vi "tsc-Show Control Settings--dialog.vi"(10 "VI Refnum":refnum<vi>) -> ()   [LabVIEW 2021]
doc: "This VI will be the user interface function for the Quick Drop action - it will list all controls on the front panel along with their UI Theme Levels and Boolean Types. This will be populated before showing its front panel and will give the user faster access to edit all controls on the front panel.\n\n->If there are any changes made and \"Apply\" is selected, it will apply the updated tags and save the VI\n->If Cancel is selected, the updates made will not be implemented\n\n<b>Code Developed By:</b>\nTechnology Service Corporation\n1983 S Liberty Drive\nBloomington, IN 47403\nPhone: 812 558-7100\nwww.tsc.com/atcs\n\nDeveloper:\nDaniel Coons"
uses:
  <vilib>/Utility/traverseref.llb/VI Scripting - Traverse.lvlib
  <vilib>/Utility/traverseref.llb/TRef TravTarget.ctl
  control info.ctl
  user32.dll
panel:
  out "header":bool
  in  "Cancel":bool
  in  "Apply":bool
  in  "control info":T1[](array[typedef]) {"Boolean Type" items=["Undefined", "N/A", "Outline", "No-Outline", "Tonal", "Filled", "Transparent", "FAB", "Elevated"]; "UI Theme Level" items=["Undefined", "N/A", "Primary", "Secondary", "Tertiary", "Error", "Primary Fixed", "Secondary Fixed", "Tertiary Fixed", "Label Only", "No Change"]}
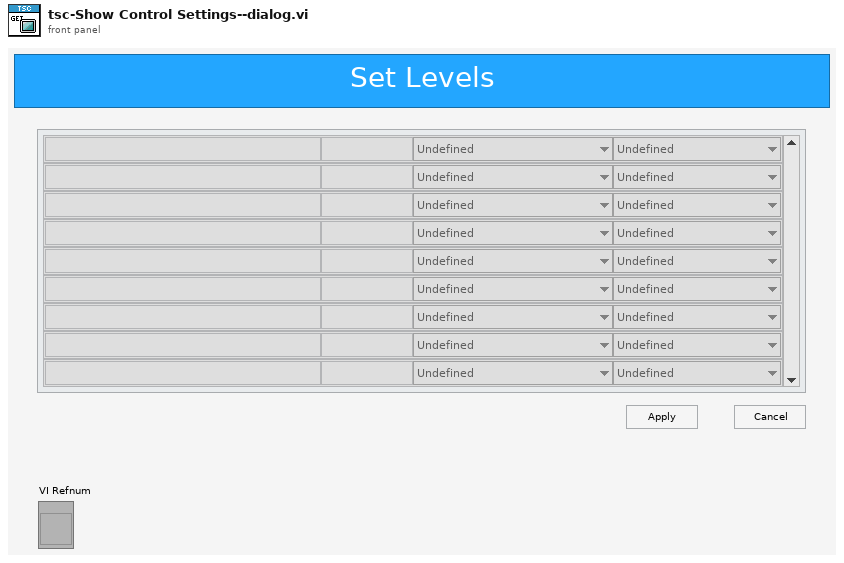
[diagram p1: front panel]
types:
  T1 = typedef "control info.ctl" = cluster{"label":string, "control type":string, "UI Theme Level":u16, "Boolean Type":u16}
  T2 = typedef "TRef TravTarget.ctl" = enum16{"FP", "BD", "Other"}
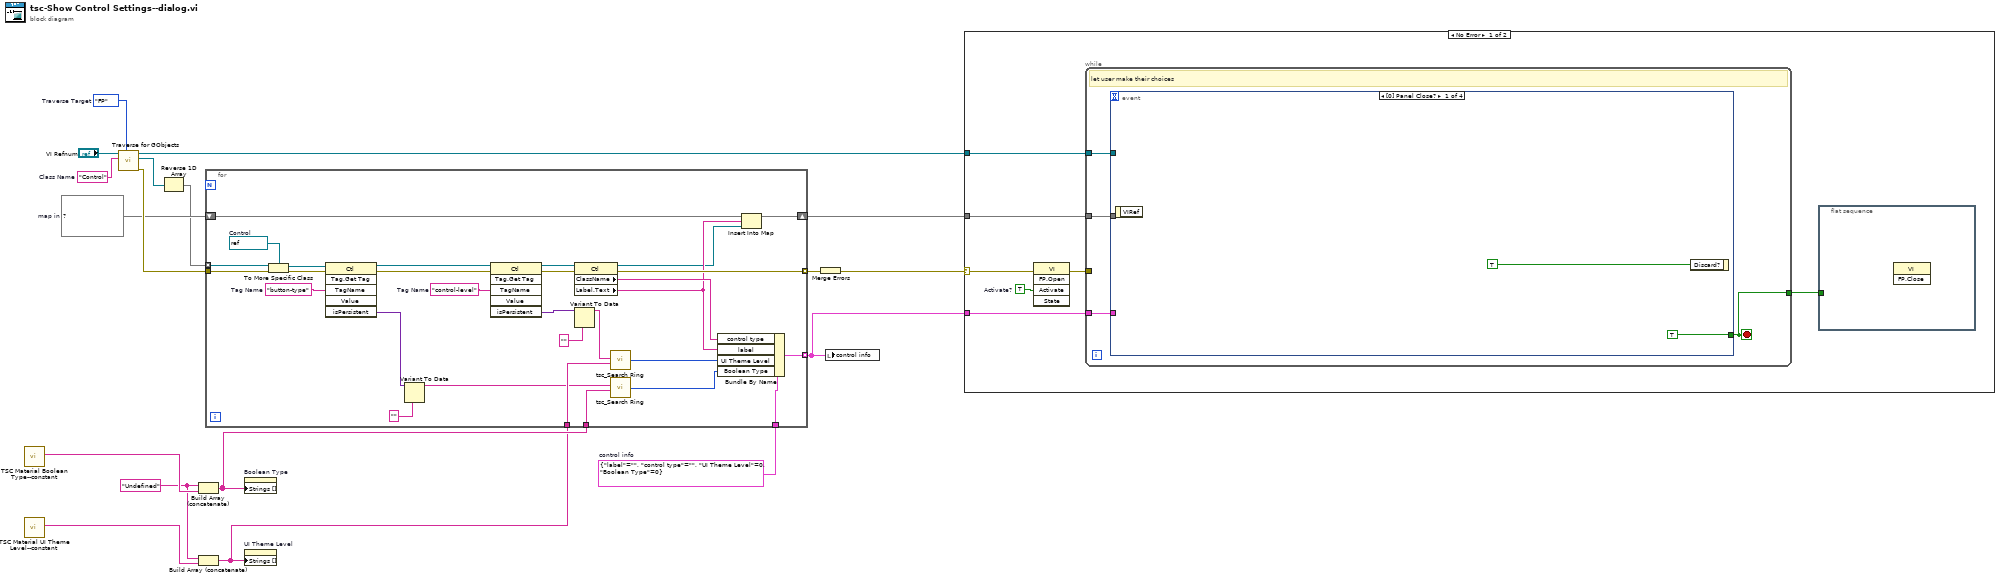
[diagram p0: block diagram]
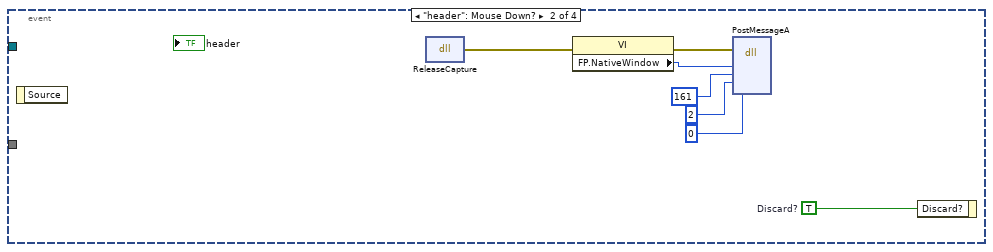
[diagram p2: hidden frame]
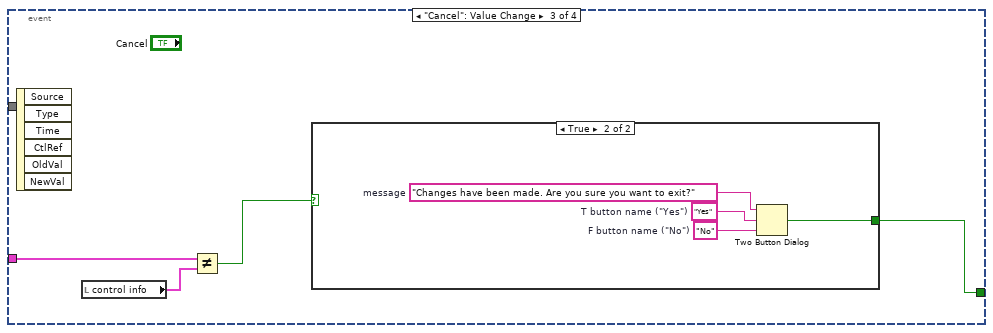
[diagram p3: hidden frame]
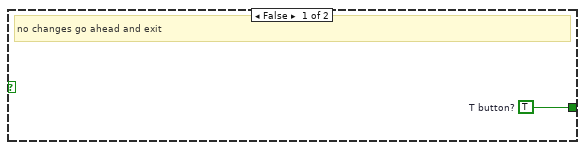
[diagram p4: hidden frame]
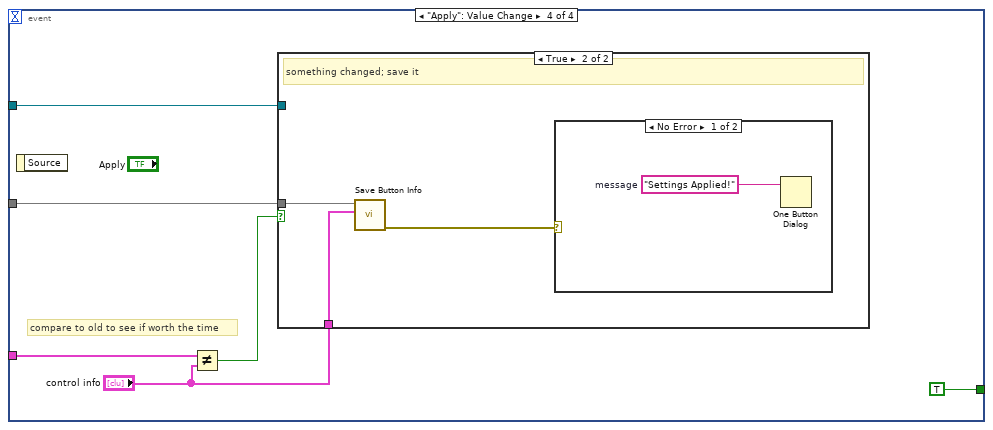
[diagram p5: hidden frame]
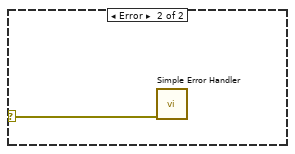
[diagram p7: hidden frame]
diagram:
  w5 = "Undefined"
  w10 = map{string, refnum<vi>} {}  # map in
  w13 = T1 {"label"="", "control type"="", "UI Theme Level"=0, "Boolean Type"=0}  # control info
  w17 = TRef_TravTarget."FP"  # Traverse Target
  w18 = "Control"  # Class Name
  n1 = call "TSC Material Boolean Type--constant.vi"() -> ("boolean types"=w12:string[])  [unwired: 11 in]
  n2 = call "TSC Material UI Theme Level--constant.vi"() -> ("UI theme levels"=w3:string[])  [unwired: 11 in]
  n3 = call <vilib>:"Traverse for GObjects.vi"("Traverse Target"=w17, "Class Name"=w18, "VI Refnum"="VI Refnum") -> ("error out"=w15:errorcluster, "References"=w16:refnum<vi>[], "dup VI Refnum"=w7:refnum<vi>)  [unwired: 5 in, 1 out]
  n4 = Reverse 1D Array(array=w16) -> (reversed array=w1:refnum<vi>[])
  n5 = Build Array (concatenate)(w5, w12) -> (w4:string[])
  n6 = Build Array (concatenate)(w5, w3) -> (w2:string[])
  n7 = for {
    tunnel: w1 -> [w34] mode=indexing
    tunnel: w15 -> [w44]
    tunnel: [w37] -> w14 mode=indexing
    tunnel: w13 -> [w31]
    tunnel: w4 -> [w21]
    tunnel: [w29] -> w11 mode=indexing
    tunnel: w2 -> [w24]
    shift-right: [w27] -> w9
    shift-left: w10 -> [w28]
    w32 = refnum<vi> refnum  # Control
    w38 = "control-level"  # Tag Name
    w47 = "button-type"  # Tag Name
    n8 = To More Specific Class(target class=w32, reference=w34, error in=w44) -> (specific class reference=w33:refnum<vi>, error out=w35:errorcluster)
    n9 = invoke class="Ctl" method="Tag.Get Tag"(reference=w33, error in=w35, "TagName"=w47) -> (reference out=w41:refnum<vi>, error out=w43:errorcluster, "isPersistent"=w46:variant)  [unwired: 3 in, 3 out]
    n10 = Variant To Data(type="", Variant=w46) -> (data=w20:string)  [unwired: 1 in, 1 out]
    n11 = invoke class="Ctl" method="Tag.Get Tag"(reference=w41, error in=w43, "TagName"=w38) -> (reference out=w36:refnum<vi>, error out=w42:errorcluster, "isPersistent"=w39:variant)  [unwired: 3 in, 3 out]
    n12 = property class="Ctl"(reference=w36, error in=w42) -> (reference out=w25:refnum<vi>, error out=w37:errorcluster, "ClassName"=w30:string, "Label.Text"=w26:string)
    n13 = Variant To Data(type="", Variant=w39) -> (data=w23:string)  [unwired: 1 in, 1 out]
    n14 = call "tsc_Search Ring.vi"("Values"=w24, "Search Item"=w23) -> ("Index"=w22:u16)  [unwired: 2 in]
    n15 = call "tsc_Search Ring.vi"("Values"=w21, "Search Item"=w20) -> ("Index"=w19:u16)  [unwired: 2 in]
    n16 = Bundle By Name(cluster=w31, "control type"=w30, "label"=w26, "UI Theme Level"=w22, "Boolean Type"=w19) -> (w29:T1)
    n17 = Insert Into Map(map in=w28, key=w26, value=w25) -> (map out=w27:map{string, refnum<vi>})  [unwired: 2 out]
  }
  n18 = property on="Boolean Type" class="Ring (strict)"("Strings []"=w4) -> ()  [unwired: 2 in, 2 out]
  n19 = property on="UI Theme Level" class="Ring (strict)"("Strings []"=w2) -> ()  [unwired: 2 in, 2 out]
  n20 = Merge Errors(w14) -> (w8:errorcluster)
  n21 = local write "control info"(w11) -> ()
  n22 = case shown="No Error" w8 {
    selector: w8 -> [w52 _]
    tunnel: w11 -> [w54 _]
    tunnel: w9 -> [w53 _]
    tunnel: w7 -> [w48 _]
    frame No Error {
      w51 = TRUE  # Activate?
      n23 = invoke class="VI" method="FP.Open"(error in=w52, "Activate"=w51) -> (error out=w50:errorcluster)  [unwired: 3 in, 4 out]
      n24 = while {
        tunnel: w54 -> [w58]
        tunnel: w53 -> [w57]
        tunnel: w50 -> [_]
        tunnel: w48 -> [w56]
        tunnel: [w55] -> w49
        stop <- w55 stop-if-true
        # "let user make their choices"
        n25 = event shown="[0] Panel Close?" {
          selector: _ -> [_ _ _ _]
          dyn-events: _ -> [_ _ _ _]
          timeout: _ -> [_ _ _ _]
          tunnel: [TRUE _ w68 TRUE] -> w55
          tunnel: w58 -> [_ _ w71 w81]
          tunnel: w57 -> [_ _ _ w80]
          tunnel: w56 -> [_ _ _ w77]
          event Panel Close? {
            n26 = event-data() -> ()  [unwired: 1 in, 1 out]
            n27 = event-data("Discard?"=TRUE) -> ()  [unwired: 1 in, 1 out]
          }
          event "header": Mouse Down? {
            w61 = TRUE  # Discard?
            n28 = event-data() -> ()  [unwired: 1 in, 1 out]
            n29 = dll-call lib="user32.dll" fn="ReleaseCapture"() -> (error out=w64:errorcluster)  [unwired: 4 in, 1 out]
            n30 = property class="VI"(error in=w64) -> (error out=w63:errorcluster, "FP.NativeWindow"=w62:u64)  [unwired: 1 in, 1 out]
            n31 = dll-call lib="user32.dll" fn="PostMessageA"(error in=w63, "hWnd"=w62, "Msg"=161, "wParam"=2, "lParam"=0) -> ()  [unwired: 7 in, 2 out]
            n32 = event-data("Discard?"=w61) -> ()  [unwired: 1 in, 1 out]
          }
          event "Cancel": Value Change {
            n33 = event-data() -> ()  [unwired: 1 in, 6 out]
            n34 = local read "control info"() -> (w70:T1[])
            n35 = Not Equal?(x=w71, y=w70) -> (x != y?=w69:bool)
            n36 = case shown="True" w69 {
              tunnel: [w72 w73] -> w68
              frame False {
                w72 = TRUE  # T button?
                # "no changes go ahead and exit"
              }
              frame True {
                w76 = "No"  # F button name ("No")
                w75 = "Yes"  # T button name ("Yes")
                w74 = "Changes have been made. Are you sure you want to exit?"  # message
                n37 = Two Button Dialog(message=w74, 1:w76, 2:w75) -> (T button?=w73:bool)
              }
            }
          }
          event "Apply": Value Change {
            # "compare to old to see if worth the time"
            n38 = event-data() -> ()  [unwired: 1 in, 1 out]
            n39 = Not Equal?(x=w81, y="control info") -> (x != y?=w78:bool)
            n40 = case shown="True" w78 {
              tunnel: w80 -> [_ w85]
              tunnel: "control info" -> [_ w84]
              tunnel: w77 -> [_ _]
              frame False {
              }
              frame True {
                # "something changed; save it"
                n41 = call "Save Button Info.vi"("control info"=w84, "map in"=w85) -> ("error out"=w83:errorcluster)  [unwired: 9 in]
                n42 = case shown="No Error" w83 {
                  selector: w83 -> [_ w87]
                  frame No Error {
                    w86 = "Settings Applied!"  # message
                    n43 = One Button Dialog(message=w86) -> ()  [unwired: 1 in, 1 out]
                  }
                  frame Error {
                    n44 = call <vilib>:"Simple Error Handler.vi"("error in (no error)"=w87) -> ()  [unwired: 4 in, 5 out]
                  }
                }
              }
            }
          }
        }
      }
      n45 = flat-sequence {
        tunnel: w49 -> [_]
        frame #0 {
          n46 = invoke class="VI" method="FP.Close"() -> ()  [unwired: 3 in, 3 out]
        }
      }
    }
    frame Error {
    }
  }
